vi "REP(HB).vi"() -> ()   [LabVIEW 2014]
uses:
  <vilib>/addons/zeromq/socket_type.ctl
  <vilib>/addons/zeromq/zmq_context.lvclass
  <vilib>/addons/zeromq/zeromq.lvlib
  <vilib>/addons/zeromq/zmq_socket.lvclass
panel:
  out "connected":bool
  in  "stop":bool
  out "last message":timestamp
  out "concatenated string":string
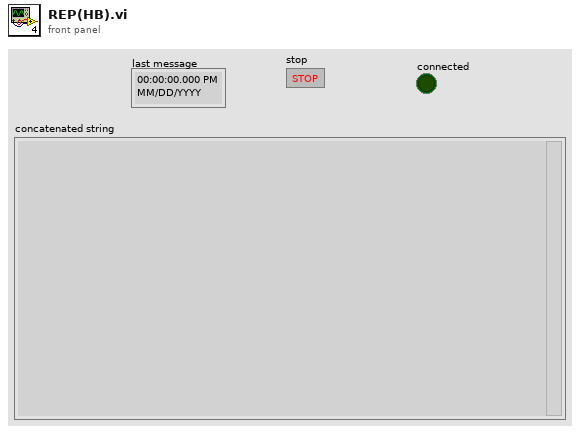
[diagram p1: front panel]
types:
  T1 = typedef "zeromq.lvlib/socket_type.ctl" = enum8{"ZMQ_PAIR", "ZMQ_PUB", "ZMQ_SUB", "ZMQ_REQ", "ZMQ_REP", "ZMQ_DEALER", "ZMQ_ROUTER", "ZMQ_PULL", "ZMQ_PUSH", "ZMQ_XPUB", "ZMQ_XSUB", "ZMQ_STREAM", "ZMQ_SERVER", "ZMQ_CLIENT", "ZMQ_RADIO", "ZMQ_DISH", "ZMQ_GATHER", "ZMQ_SCATTER", "ZMQ_DGRAM"}
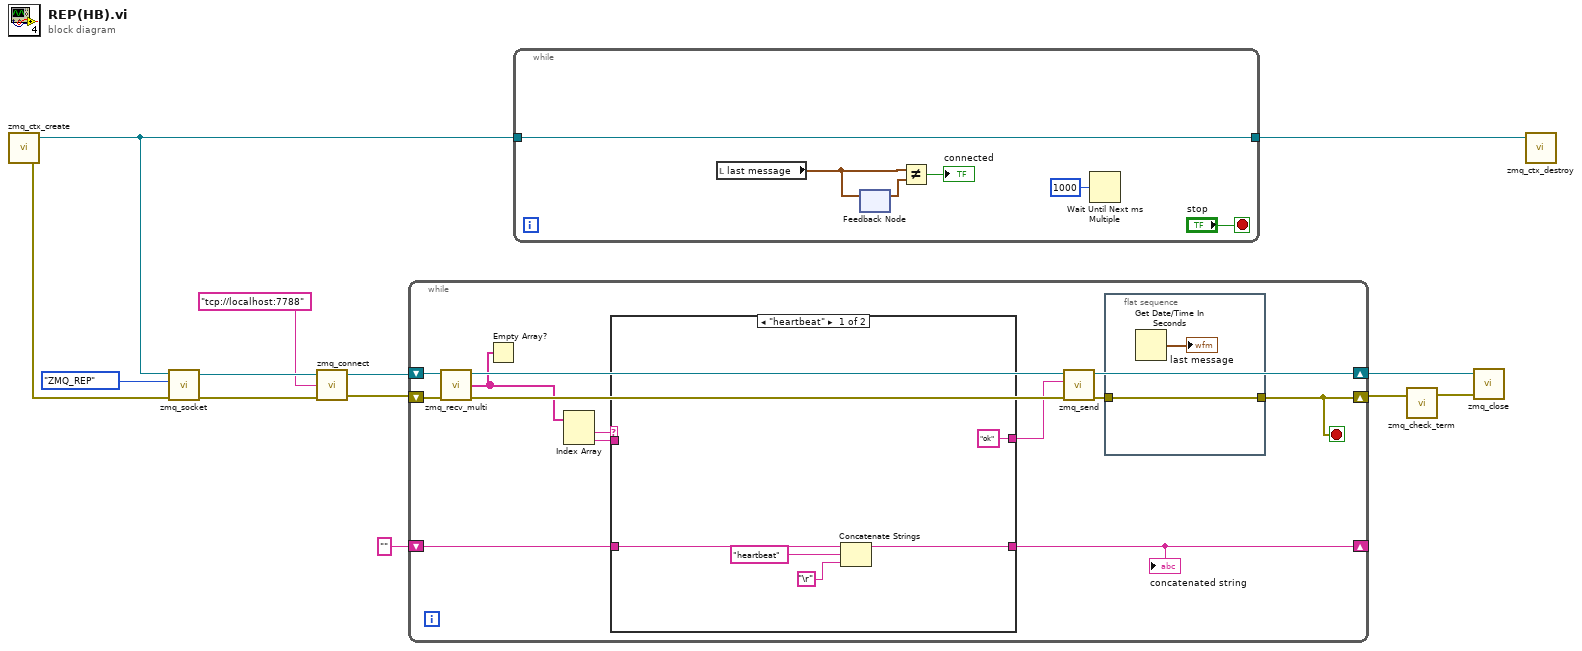
[diagram p0: block diagram]
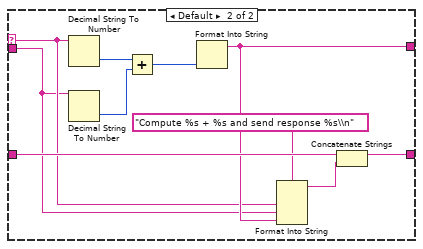
[diagram p2: hidden frame]
diagram:
  n1 = call <vilib>:"zmq_ctx_create.vi"() -> ("error out"=w12:errorcluster, "context out"=w1:refnum<class "zmq_context.lvclass">)  [unwired: 4 in]
  n2 = call <vilib>:"zmq_socket.vi"("error in"=w12, "socket type"=socket_type."ZMQ_REP", "context in"=w1) -> ("error out"=w10:errorcluster, "socket out"=w11:refnum<class "zmq_socket.lvclass">)  [unwired: 2 in, 1 out]
  n3 = call <vilib>:"zmq_connect.vi"("error in"=w10, "endpoint"="tcp://localhost:7788", "socket in"=w11) -> ("error out"=w7:errorcluster, "socket out"=w8:refnum<class "zmq_socket.lvclass">)  [unwired: 1 in]
  n4 = while {
    shift-right: [w22] -> w6
    shift-left: w8 -> [w26]
    shift-right: [w17] -> w4
    shift-left: w7 -> [w25]
    shift-right: [w19] -> _
    shift-left: "" -> [w21]
    stop <- w17 stop-if-true
    n5 = call <vilib>:"zmq_recv_multi.vi"("error in"=w25, "socket in"=w26) -> ("error out"=w23:errorcluster, "parts"=w16:string[], "socket out"=w24:refnum<class "zmq_socket.lvclass">)  [unwired: 1 in]
    n6 = Empty Array?(array=w16) -> ()  [unwired: 1 out]
    n7 = Index Array(array=w16) -> (element #1=w15:string, element #2=w14:string)  [unwired: 2 in]
    n8 = case shown="\"heartbeat\"" w15 {
      selector: w15 -> [_ w35]
      tunnel: w21 -> [w31 w41]
      tunnel: ["ok" w40] -> w20
      tunnel: [w29 w39] -> w19
      tunnel: w14 -> [_ w34]
      frame "heartbeat" {
        n9 = Concatenate Strings(w31, "heartbeat" ("string"), "\r") -> (w29:string)
      }
      frame Default {
        n10 = Decimal String To Number(string=w35) -> (number=w38:i32)  [unwired: 2 in, 1 out]
        n11 = Decimal String To Number(string=w34) -> (number=w37:i32)  [unwired: 2 in, 1 out]
        n12 = Add(x=w38, y=w37) -> (x+y=w36:i32)
        n13 = Format Into String(w36) -> (resulting string=w40:string)  [unwired: 3 in, 1 out]
        n14 = Format Into String(format string="Compute %s + %s and send response %s\\n", w35, w34, w40) -> (resulting string=w32:string)  [unwired: 2 in, 1 out]
        n15 = Concatenate Strings(w41, w32) -> (w39:string)
      }
    }
    "concatenated string" <- w19
    n16 = call <vilib>:"zmq_send.vi"("error in"=w23, "data"=w20, "socket in"=w24) -> ("error out"=w18:errorcluster, "socket out"=w22:refnum<class "zmq_socket.lvclass">)  [unwired: 4 in]
    n17 = flat-sequence {
      tunnel: [w42] -> w17
      tunnel: w18 -> [w42]
      frame #0 {
        n18 = Get Date/Time In Seconds() -> (seconds since 1Jan1904=→"last message":timestamp)
      }
    }
  }
  n19 = while {
    tunnel: [w49] -> w2
    tunnel: w1 -> [w49]
    stop <- "stop" stop-if-true
    n20 = local read "last message"() -> (w46:timestamp)
    n21 = feedback-in #1(w46) -> ()
    n22 = feedback #1() -> (w45:timestamp)  [unwired: 1 in]
    n23 = Not Equal?(x=w46, y=w45) -> (x != y?=→"connected":bool)
    n24 = Wait Until Next ms Multiple(millisecond multiple=u32 1000) -> ()  [unwired: 1 out]
  }
  n25 = call <vilib>:"zmq_check_term.vi"("error in"=w4) -> ("error out"=w3:errorcluster)  [unwired: 1 in, 1 out]
  n26 = call <vilib>:"zmq_close.vi"("error in"=w3, "socket"=w6) -> ()  [unwired: 3 in, 1 out]
  n27 = call <vilib>:"zmq_ctx_destroy.vi"("context in"=w2) -> ()  [unwired: 4 in, 1 out]
